vi "Get Channels.vi"(8 "error in (no error)":errorcluster {"code" format="%.0x"}, 9 "ValBufferSize":i32=2048, 11 "instrument handle":refnum<k15>) -> (0 "error out":errorcluster {"code" format="%.0x"}, 1 "ValActualSize":i32, 2 "Val":i32[](array[numeric]), 3 "instrument handle out":refnum<k15>)   [LabVIEW 2014, in "Agilent NA.lvlib"]
doc: "Get channels to be calibrated."
uses:
  Agilent NA.lvlib
  AgNA.dll
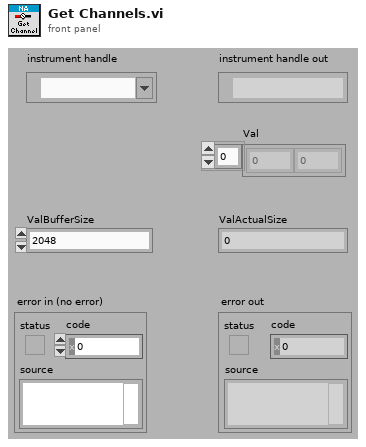
[diagram p1: front panel]
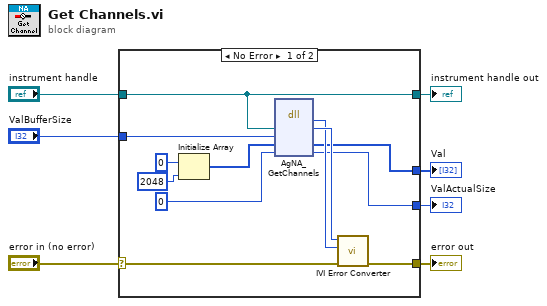
[diagram p0: block diagram]
diagram:
  n1 = case shown="No Error" "error in (no error)" {
    selector: "error in (no error)" -> [w17 w21]
    tunnel: [w16 w21] -> w7
    tunnel: "ValBufferSize" -> [w15 _]
    tunnel: [w11 _] -> w4
    tunnel: [w9 _] -> w3
    tunnel: "instrument handle" -> [w8 w20]
    tunnel: [w8 w20] -> w1
    frame No Error {
      n2 = Initialize Array(0 ("element"), 2048 ("dimension size")) -> (w14:i32[])
      n3 = dll-call lib="AgNA**.dll" fn="AgNA_GetChannels"("Vi"=w8, "ValBufferSize"=w15, "Val"=w14, "ValActualSize"=0) -> (w18:i32, "Vi"=w19:u32, "Val"=w11:i32[], "ValActualSize"=w9:i32)  [unwired: 4 in, 2 out]
      n4 = call "IVI Error Converter.vi"("error in (no error)"=w17, "IVI error code (0)"=w18, "instrument handle"=w19) -> ("error out"=w16:errorcluster)  [unwired: 7 in, 1 out]
    }
    frame Error {
    }
  }
  "error out" <- w7
  "instrument handle out" <- w1
  "Val" <- w4
  "ValActualSize" <- w3
